vi "Patch data export-Initialise all.vi"(7 "Output file path":path=path "C:/Users/Teo/Desktop/UCL Datasets/160915_13_48_57 FunctAcq-6 patches", 9 "Peak value in dataset (I16)":dbl=4000.0 format="%#_13g", 10 "8-bit Image refs cluster":T1, 11 "Cursors location":T3) -> (0 "error out":errorcluster, 3 "U8 Image ref":T2)   [LabVIEW 2017]
uses:
  <vilib>/vision/Image Controls.llb/IMAQ Image.ctl
  User Interface/Visualisation/Patch-Vol video generator/Typedefs/8bit sync-IMAQ image refs.ctl
  User Interface/Visualisation/Patch-Vol video generator/Globals/gl_8-bit montage window ctrl refs.vi
  User Interface/Visualisation/Timelapse Viewer/Globals/gl_Time series viewer globals.vi
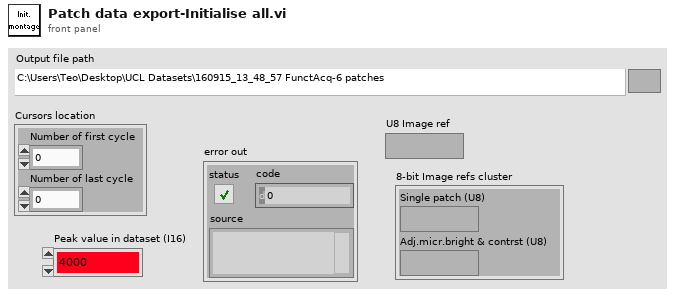
[diagram p1: front panel]
types:
  T1 = typedef "8bit sync-IMAQ image refs.ctl" = cluster{"Single patch (U8)":T2, "Adj.micr.bright & contrst (U8)":T2}
  T2 = typedef "IMAQ Image.ctl" = refnum<image>
  T3 = cluster{"Number of first cycle":i32, "Number of last cycle":i32}
  T4 = typedef "8-bit video export window ctrl refs.ctl" = cluster{"This VI":refnum<vi>, "Add speed data":refnum<vi>, "Add camera videos":refnum<vi>, "Stop button":refnum<vi>, "Camera Video Adjustments":refnum<vi>, "Microscope Image Adjustments":refnum<vi>, "Execute":refnum<vi>, "Codec":refnum<vi>, "Channel to load":refnum<vi>, "Speed graph behaviour":refnum<vi>, "Include speed graph":refnum<vi>, "Number of rows to generate":refnum<vi>, "Path":refnum<vi>}
  T5 = typedef "AVI playback header info cluster.ctl" = cluster{"Frame Size":u32, "AOD fill time (us)":dbl, "Dwell time (us)":dbl, "Frame period (ms)":dbl, "Number of Miniscans":u16, "Number of Pixels in Miniscan":u16}
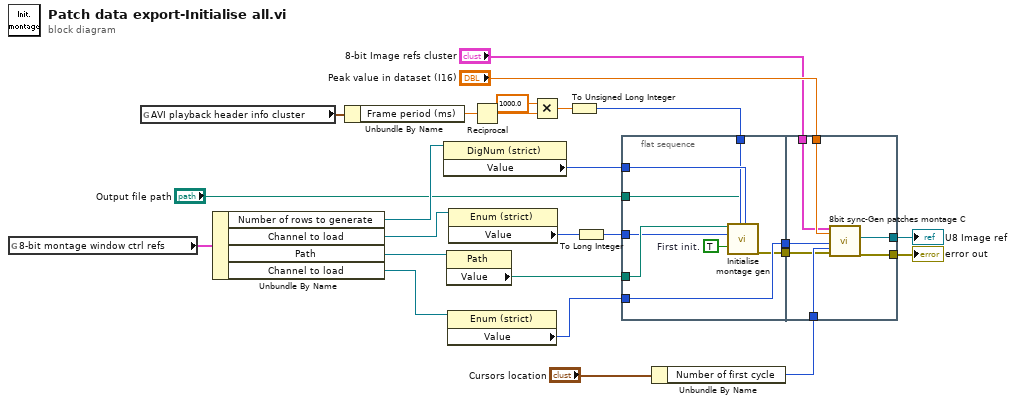
[diagram p0: block diagram]
diagram:
  n1 = global read "gl_8-bit montage window ctrl refs.vi" "8-bit montage window ctrl refs"() -> (w17:T4)
  n2 = global read "gl_Time series viewer globals.vi" "AVI playback header info cluster"() -> (w13:T5)
  n3 = Unbundle By Name(w17) -> ("Number of rows to generate"=w23:refnum<vi>, "Channel to load"=w16:refnum<vi>, "Path"=w21:refnum<vi>, "Channel to load"=w25:refnum<vi>)
  n4 = Unbundle By Name(w13) -> ("Frame period (ms)"=w12:dbl)
  n5 = property class="DigNum (strict)"(reference=w23) -> ("Value"=w24:i32)  [unwired: 1 in, 2 out]
  n6 = property class="Path"(reference=w21) -> ("Value"=w22:path)  [unwired: 1 in, 2 out]
  n7 = property class="Enum (strict)"(reference=w25) -> ("Value"=w6:enum16{"Green", "Red"})  [unwired: 1 in, 2 out]
  n8 = property class="Enum (strict)"(reference=w16) -> ("Value"=w15:enum16{"Green", "Red"})  [unwired: 1 in, 2 out]
  n9 = Reciprocal(x=w12) -> (1/x=w11:dbl)
  n10 = Multiply(x=1000.0, y=w11) -> (x*y=w10:dbl)
  n11 = To Unsigned Long Integer(number=w10) -> (unsigned 32bit integer=w8:u32)
  n12 = To Long Integer(number=w15) -> (32bit integer=w14:i32)
  n13 = flat-sequence {
    tunnel: w24 -> [w32]
    tunnel: w22 -> [w33]
    tunnel: w14 -> [w31]
    tunnel: w8 -> [w30]
    tunnel: [w29] -> w7
    tunnel: w6 -> [w29]
    tunnel: [w28] -> w4
    tunnel: "Output file path" -> [w27]
    tunnel: w18 -> [w40]
    tunnel: [w38] -> w20
    tunnel: w7 -> [w39]
    tunnel: [w37] -> w5
    tunnel: w4 -> [w36]
    tunnel: "Peak value in dataset (I16)" -> [w35]
    tunnel: "8-bit Image refs cluster" -> [w34]
    frame #0 {
      w26 = TRUE  # First init.
      n14 = call "Initialise montage gen.vi"("ExperimentPath"=w33, "Channel"=w31, "First init."=w26, "Output file path"=w27, "Frames Per Second"=w30, "Number of rows to generate"=w32) -> ("error out"=w28:errorcluster)  [unwired: 10 in, 3 out]
    }
    frame #1 {
      n15 = call "8bit sync-Gen patches montage C.vi"("8-bit Image refs cluster"=w34, "max value"=w35, "Channel"=w39, "Global cycle number among all trials"=w40, "error in (no error)"=w36) -> ("U8 Image (Montage)"=w38:T2, "error out"=w37:errorcluster)  [unwired: 13 in]
    }
  }
  n16 = Unbundle By Name("Cursors location") -> ("Number of first cycle"=w18:i32)
  "U8 Image ref" <- w20
  "error out" <- w5
